vi "set channel property.vi"(8 "error in":errorcluster, 9 "value":string, 10 "property":string, 11 "channel in":refnum<class "TBM channel.lvclass">) -> (0 "error out":errorcluster, 3 "channel out":refnum<class "TBM channel.lvclass">)   [LabVIEW 2013, in "TBM channel.lvclass"]
uses:
  TBM channel.lvclass
  <vilib>/NI/Tag Bus/tag/tag descriptor.lvclass/tag descriptor.ctl
  <vilib>/NI/Tag Bus/tag/Data Type.ctl
  channel classification.ctl
  TBM channel.lvclass/TBM channel.ctl
  <vilib>/NI/Tag Bus/tag/tag descriptor.lvclass
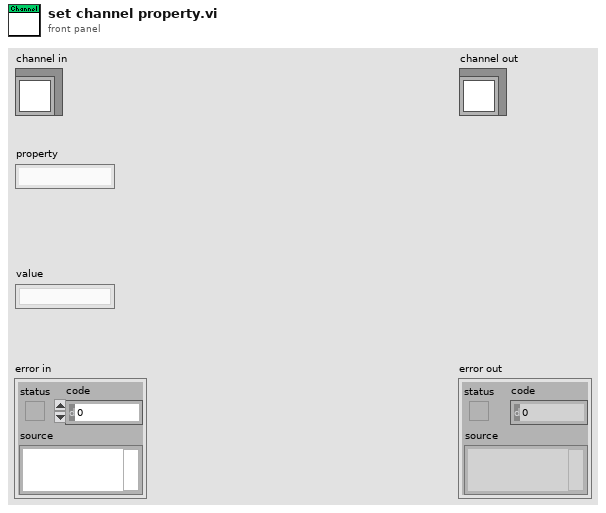
[diagram p1: front panel]
types:
  T1 = typedef "tag bus.lvlib/tag descriptor.lvclass/Data Type.ctl" = enum16{"Double", "Single", "I64", "I32", "I16", "I8", "U64", "U32", "U16", "U8", "Boolean", "String", "Array of Double", "Array of Single", "Array of I64", "Array of I32", "Array of I16", "Array of I8", "Array of U64", "Array of U32", "Array of U16", "Array of U8", "Array of Boolean", "Array of String"}
  T2 = typedef "TBM channel.lvclass/channel classification.ctl" = enum16{"input data", "output data", "processing parameter", "processing result"}
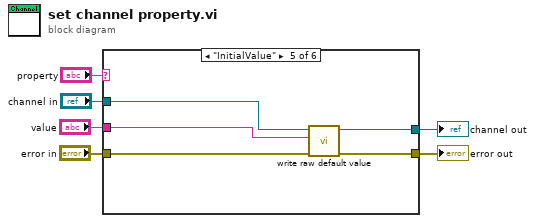
[diagram p0: block diagram]
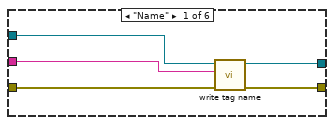
[diagram p2: hidden frame]
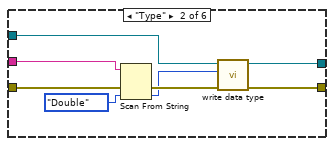
[diagram p3: hidden frame]
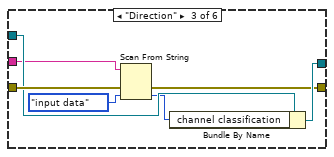
[diagram p4: hidden frame]
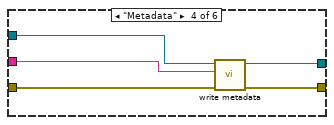
[diagram p5: hidden frame]
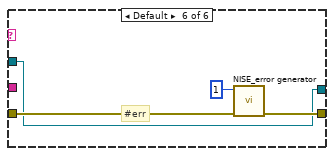
[diagram p6: hidden frame]
diagram:
  n1 = case shown="\"InitialValue\"" "property" {
    tunnel: [w10 w17 w23 w30 w35 w39] -> w4
    tunnel: "error in" -> [w11 w18 w26 w31 w36 w40]
    tunnel: "channel in" -> [w9 w19 w25 w29 w34 w37]
    tunnel: "value" -> [w8 w14 w20 w27 w32 _]
    tunnel: [w7 w12 w24 w28 w33 w37] -> w1
    frame "Name" {
      n2 = call <vilib>:"write tag name.vi"("error in"=w11, "name"=w8, "system tag in"=w9) -> ("error out"=w10:errorcluster, "system tag out"=w7:refnum<class "TBM channel.lvclass">)  [unwired: 7 in]
    }
    frame "Type" {
      n3 = Scan From String(input string=w14, error in=w18, default 1=Data_Type."Double" ("data type")) -> (error out=w16:errorcluster, output 1=w13:T1)  [unwired: 2 in, 2 out]
      n4 = call <vilib>:"write data type.vi"("error in"=w16, "data type"=w13, "system tag in"=w19) -> ("error out"=w17:errorcluster, "system tag out"=w12:refnum<class "TBM channel.lvclass">)  [unwired: 7 in]
    }
    frame "Direction" {
      n5 = Scan From String(input string=w20, error in=w26, default 1=channel_classification."input data" ("channel classification")) -> (error out=w23:errorcluster, output 1=w21:T2)  [unwired: 2 in, 2 out]
      n6 = Bundle By Name(cluster=w25, "channel classification"=w21) -> (w24:refnum<class "TBM channel.lvclass">)
    }
    frame "Metadata" {
      n7 = call <vilib>:"write metadata.vi"("error in"=w31, "metadata"=w27, "system tag in"=w29) -> ("error out"=w30:errorcluster, "system tag out"=w28:refnum<class "TBM channel.lvclass">)  [unwired: 7 in]
    }
    frame "InitialValue" {
      n8 = call <vilib>:"write raw default value.vi"("error in"=w36, "raw default"=w32, "system tag in"=w34) -> ("error out"=w35:errorcluster, "system tag out"=w33:refnum<class "TBM channel.lvclass">)  [unwired: 7 in]
    }
    frame Default {
      # "#err"
      n9 = call <vilib>:"NISE_error generator.vi"("error in"=w40, "error code (0)"=1) -> ("error out"=w39:errorcluster)  [unwired: 7 in]
    }
  }
  "error out" <- w4
  "channel out" <- w1
